vi "In Place Read Scalar I32.vi"(8 "error in (no error)":errorcluster, 10 "value in":i32, 11 "pointer in":u64) -> (0 "error out":errorcluster, 2 "value out":i32, 3 "pointer out":u64)   [LabVIEW 2013, in "Linux RT IPC.Shared Memory.lvlib"]
uses:
  Linux RT IPC.Shared Memory.lvlib
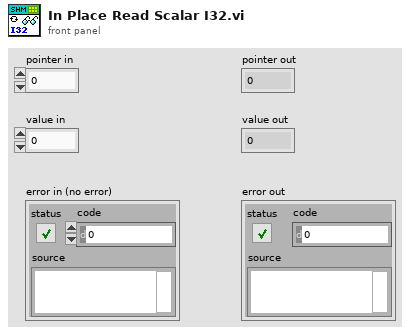
[diagram p1: front panel]
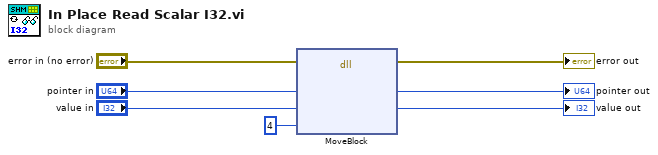
[diagram p0: block diagram]
diagram:
  n1 = dll-call lib="LabVIEW" fn="MoveBlock"(error in="error in (no error)", "pointer"="pointer in", "data"="value in", "size"=u64 4) -> (error out=→"error out":errorcluster, "pointer"=→"pointer out":u64, "data"=→"value out":i32)  [unwired: 4 in, 1 out]
